vi "WLAN_STF_&_LTF.vi"() -> (3 "STF & LTF":cdb[](array[numeric]))   [LabVIEW 2022 SP3]
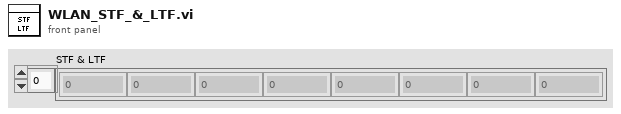
[diagram p1: front panel]
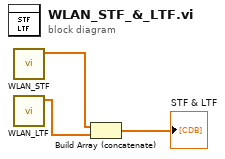
[diagram p0: block diagram]
diagram:
  n1 = call "WLAN_STF.vi"() -> ("STF"=w3:cdb[])  [unwired: 11 in]
  n2 = call "WLAN_LTF.vi"() -> ("LTF"=w1:cdb[])  [unwired: 11 in]
  n3 = Build Array (concatenate)(w3, w1) -> (→"STF & LTF":cdb[])
